vi "quiz2.vi"() -> ()   [LabVIEW 2019]
panel:
  in  "stop":bool
  out "XY Graph":cluster{dbl[], dbl[]}(graph)
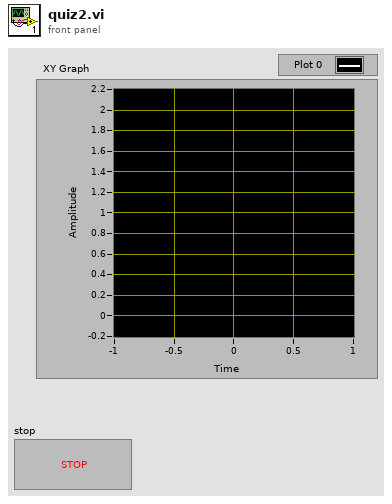
[diagram p1: front panel]
types:
  T1 = enum16{"open", "replace", "create", "open or create", "replace or create", "replace or create with confirmation"}
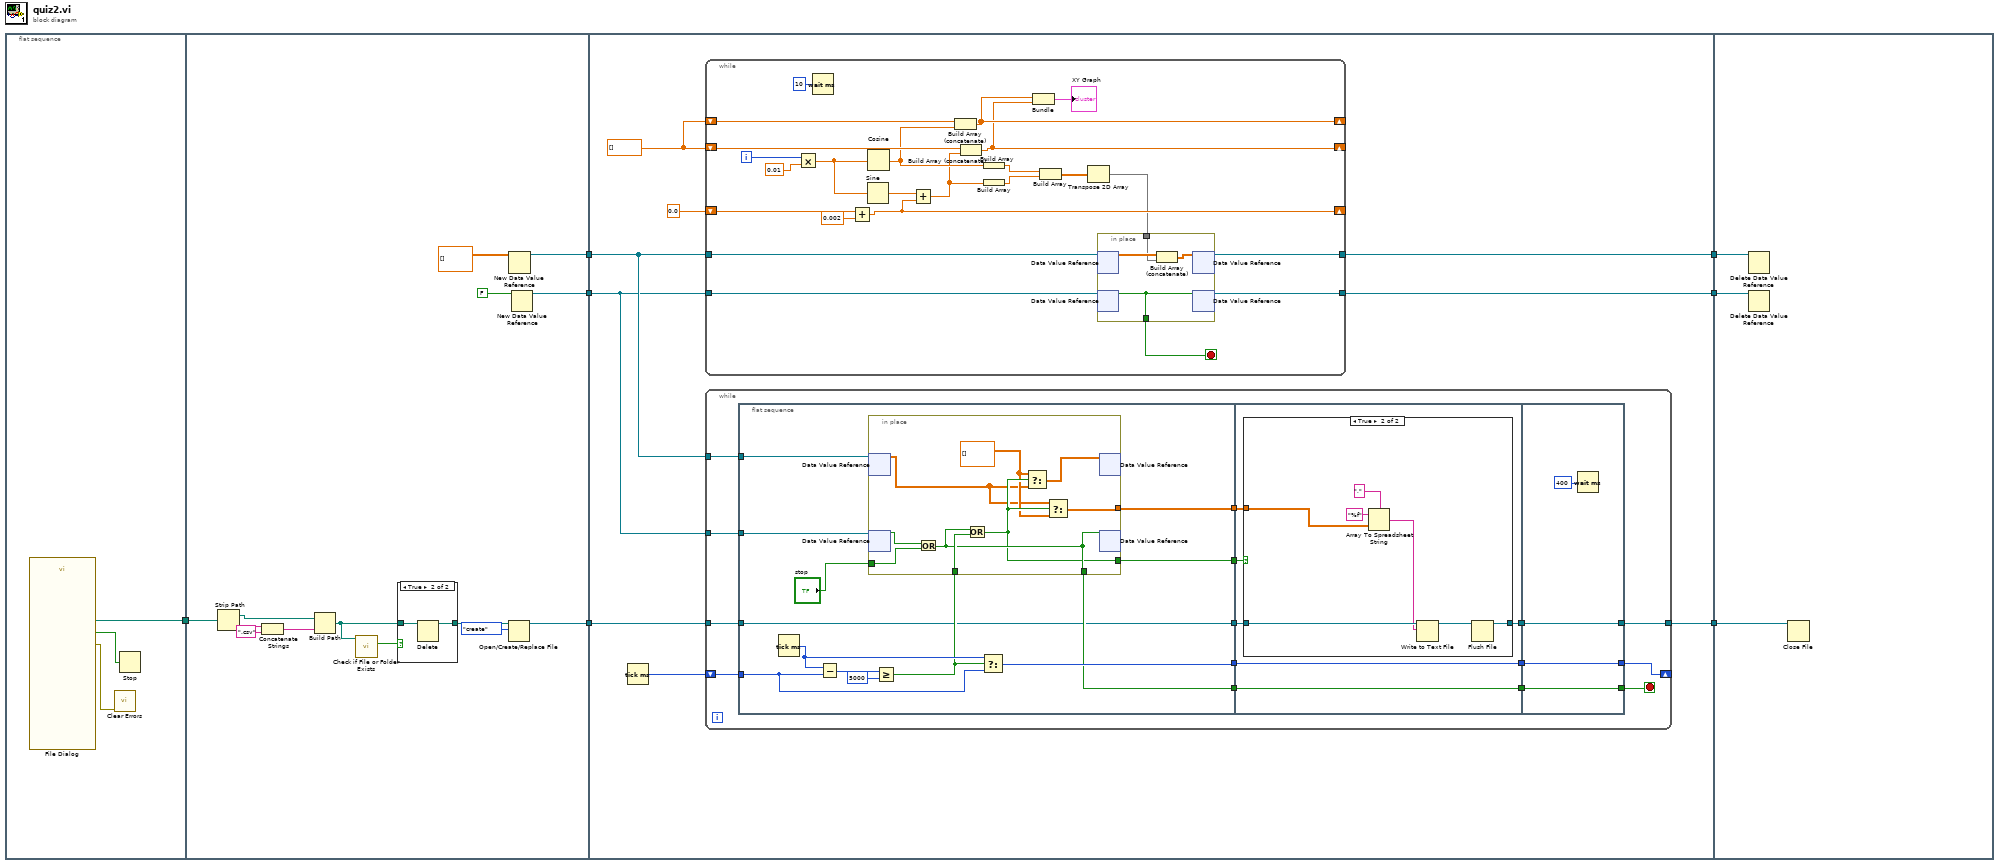
[diagram p0: block diagram]
diagram:
  n1 = flat-sequence {
    tunnel: [w8] -> w7
    tunnel: w7 -> [w24]
    tunnel: [w15] -> w6
    tunnel: [w12] -> w5
    tunnel: [w11] -> w4
    tunnel: w6 -> [w31]
    tunnel: w5 -> [w34]
    tunnel: w4 -> [w32]
    tunnel: [w30] -> w3
    tunnel: [w29] -> w2
    tunnel: [w28] -> w1
    tunnel: w3 -> [w122]
    tunnel: w2 -> [w121]
    tunnel: w1 -> [w120]
    frame #0 {
      n2 = call "File Dialog"() -> ("selected path"=w8:path, "cancelled"=w9:bool, "error out"=w10:errorcluster)  [unwired: 12 in, 1 out]
      n3 = call <vilib>:"Clear Errors.vi"("error in (no error)"=w10) -> ()  [unwired: 5 in, 2 out]
      n4 = Stop(stop? (T)=w9) -> ()
    }
    frame #1 {
      n5 = Strip Path(path=w24) -> (stripped path=w20:path, name=w23:string)
      n6 = Concatenate Strings(w23, ".csv" ("string")) -> (w21:string)
      n7 = Build Path(base path=w20, name or relative path=w21) -> (appended path=w18:path)
      n8 = call <vilib>:"Check if File or Folder Exists.vi"("path"=w18) -> ("file or folder exists?"=w19:bool)  [unwired: 8 in, 2 out]
      n9 = case shown="True" w19 {
        tunnel: w18 -> [w25 w27]
        tunnel: [w25 w26] -> w17
        frame False {
        }
        frame True {
          n10 = Delete(path (use dialog)=w27) -> (deleted path=w26:path)  [unwired: 4 in, 2 out]
        }
      }
      n11 = Open/Create/Replace File(file path (use dialog)=w17, operation (0:open)=T1."create") -> (refnum out=w15:refnum<file>)  [unwired: 4 in, 2 out]
      n12 = New Data Value Reference(data value=dbl[][] []) -> (data value reference=w12:refnum<data-value>)  [unwired: 1 in, 1 out]
      n13 = New Data Value Reference(data value=FALSE) -> (data value reference=w11:refnum<data-value>)  [unwired: 1 in, 1 out]
    }
    frame #2 {
      w36 = dbl[] []
      n14 = Tick Count (ms)() -> (millisecond timer value=w33:u32)
      n15 = while {
        tunnel: w34 -> [w51]
        shift-right: [w41] -> _
        shift-left: w33 -> [w50]
        tunnel: w32 -> [w48]
        tunnel: w31 -> [w40]
        tunnel: [w37] -> w30
        stop <- w43 stop-if-true
        n16 = flat-sequence {
          tunnel: w51 -> [w64]
          tunnel: w50 -> [w60]
          tunnel: [w59] -> w49
          tunnel: w48 -> [w58]
          tunnel: [w55] -> w47
          tunnel: [w54] -> w46
          tunnel: [w53] -> w45
          tunnel: w40 -> [w52]
          tunnel: [w52] -> w39
          tunnel: w49 -> [w76]
          tunnel: w47 -> [w79]
          tunnel: w46 -> [w78]
          tunnel: w45 -> [w77]
          tunnel: [w77] -> w44
          tunnel: [w76] -> w42
          tunnel: w39 -> [w75]
          tunnel: [w74] -> w38
          tunnel: [w90] -> w43
          tunnel: w44 -> [w90]
          tunnel: [w89] -> w41
          tunnel: w42 -> [w89]
          tunnel: w38 -> [w88]
          tunnel: [w88] -> w37
          frame #0 {
            n17 = Tick Count (ms)() -> (millisecond timer value=w61:u32)
            n18 = Subtract(x=w61, y=w60) -> (x-y=w63:u32)
            n19 = Greater Or Equal?(x=w63, y=u32 5000) -> (x >= y?=w56:bool)
            n20 = in-place {
              in-place-border: "stop" -> [w72]
              in-place-border: w56 -> [w71]
              in-place-border: [w70] -> w53
              in-place-border: [w68] -> w55
              in-place-border: [w65] -> w54
              w67 = dbl[][] [] ("t")
              n21 = in-place-dvr #1(w64) -> (w66:dbl[][])  [unwired: 1 out]
              n22 = in-place-dvr #2(w58) -> (w73:bool)  [unwired: 1 out]
              n23 = Or(x=w73, y=w72) -> (x .or. y?=w70:bool)
              n24 = Or(x=w70, y=w71) -> (x .or. y?=w68:bool)
              n25 = Select(t=w67, s=w68, f=w66) -> (s? t:f=w69:dbl[][])
              n26 = Select(t=w66, s=w68, f=w67) -> (s? t:f=w65:dbl[][])
              n27 = in-place-dvr #1(w69) -> ()  [unwired: 2 out]
              n28 = in-place-dvr #2(w70) -> ()  [unwired: 2 out]
            }
            n29 = Select(t=w61, s=w56, f=w60) -> (s? t:f=w59:u32)
          }
          frame #1 {
            n30 = case shown="True" w79 {
              tunnel: w78 -> [_ w81]
              tunnel: w75 -> [w80 w87]
              tunnel: [w80 w82] -> w74
              frame False {
              }
              frame True {
                n31 = Array To Spreadsheet String(delimiter (Tab)=",", array=w81, 3:"%f" ("format string")) -> (spreadsheet string=w84:string)
                n32 = Write to Text File(file (use dialog)=w87, text=w84) -> (refnum out=w83:refnum<file>)  [unwired: 2 in, 2 out]
                n33 = Flush File(refnum=w83) -> (refnum out=w82:refnum<file>)  [unwired: 1 in, 1 out]
              }
            }
          }
          frame #2 {
            n34 = Wait (ms)(milliseconds to wait=u32 400) -> ()  [unwired: 1 out]
          }
        }
      }
      n35 = while {
        shift-right: [w98] -> _
        shift-left: w36 -> [w114]
        shift-right: [w99] -> _
        shift-left: w36 -> [w113]
        shift-right: [w105] -> _
        shift-left: 0.0 -> [w108]
        tunnel: w34 -> [w104]
        tunnel: w32 -> [w103]
        tunnel: [w102] -> w29
        tunnel: [w101] -> w28
        i -> [w111]
        stop <- w100 stop-if-true
        n36 = Multiply(x=w111, y=0.01) -> (x*y=w109:dbl)
        n37 = Wait (ms)(milliseconds to wait=u32 10) -> ()  [unwired: 1 out]
        n38 = Add(x=w108, y=0.002) -> (x+y=w105:dbl)
        n39 = Sine(x=w109) -> (sin(x)=w106:dbl)
        n40 = Cosine(x=w109) -> (cos(x)=w95:dbl)
        n41 = Add(x=w106, y=w105) -> (x+y=w94:dbl)
        n42 = Build Array (concatenate)(w113, w95) -> (w99:dbl[])
        n43 = Build Array (concatenate)(w114, w94) -> (w98:dbl[])
        n44 = Build Array(w95) -> (w93:dbl[])
        n45 = Build Array(w94) -> (w92:dbl[])
        n46 = Bundle(w99, w98) -> (→"XY Graph":cluster{dbl[], dbl[]})  [unwired: 1 in]
        n47 = Build Array(w93, w92) -> (w97:dbl[][])
        n48 = Transpose 2D Array(2D array=w97) -> (transposed array=w96:dbl[][])
        n49 = in-place {
          in-place-border: [w119] -> w100
          in-place-border: w96 -> [w117]
          n50 = in-place-dvr #3(w104) -> (w118:dbl[][])  [unwired: 1 out]
          n51 = in-place-dvr #4(w103) -> (w119:bool)  [unwired: 1 out]
          n52 = Build Array (concatenate)(w118, w117) -> (w116:dbl[][])
          n53 = in-place-dvr #3(w116) -> (w102:refnum<data-value>)  [unwired: 1 out]
          n54 = in-place-dvr #4(w119) -> (w101:refnum<data-value>)  [unwired: 1 out]
        }
      }
    }
    frame #3 {
      n55 = Delete Data Value Reference(data value reference=w121) -> ()  [unwired: 1 in, 2 out]
      n56 = Delete Data Value Reference(data value reference=w120) -> ()  [unwired: 1 in, 2 out]
      n57 = Close File(refnum=w122) -> ()  [unwired: 1 in, 2 out]
    }
  }
